vi "Event_CloseRegistrationRef.vi"(6 "Event Registration Refnum in":T1, 8 "error in (no error)":errorcluster) -> (0 "error out":errorcluster)   [LabVIEW 2014, in "hse-misc.lvlib"]
doc: "Unregisters the given event registration from the HSE-Event \n\n\n____\nHAMPEL SOFTWARE ENGINEERING v0.7.0 (2018-07-16 18:12)"
uses:
  hse-misc.lvlib
  Event_GenericRegistration.ctl
  Event_GenericReference.ctl
  Event_GenericDatatype.ctl
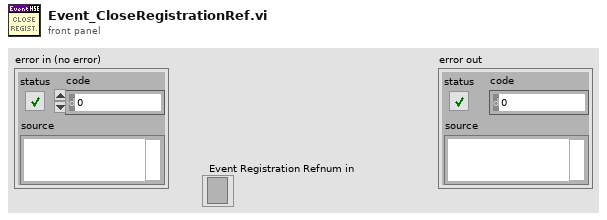
[diagram p1: front panel]
types:
  T1 = typedef "hse-misc.lvlib/Event_GenericRegistration.ctl" = refnum<event-registration>
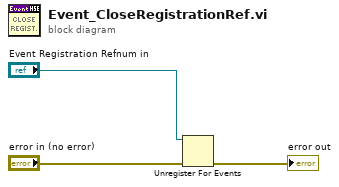
[diagram p0: block diagram]
diagram:
  n1 = Unregister For Events(event registration refnum="Event Registration Refnum in", error in="error in (no error)") -> (error out=→"error out":errorcluster)
